vi "Configure Node Info.vi"(8 "error in (no error)":errorcluster, 11 "Volatus Core in":refnum<class "Volatus Core.lvclass">) -> (0 "error out":errorcluster, 3 "Volatus Core out":refnum<class "Volatus Core.lvclass">)   [LabVIEW 2020, in "Volatus.lvlib" / "Volatus Core.lvclass"]
uses:
  Volatus Core.lvclass
  C:/dev/lv20CE/relink/lv-volatus/Volatus/Module/Module.lvclass
  Volatus Core.lvclass/Volatus Core.ctl
  Module/Module.lvclass
  lv-vecto/Vecto/Node Config/Node Config.lvclass
  C:/dev/lv20CE/relink/lv-volatus/Volatus/Volatus Core/Volatus Core.lvclass
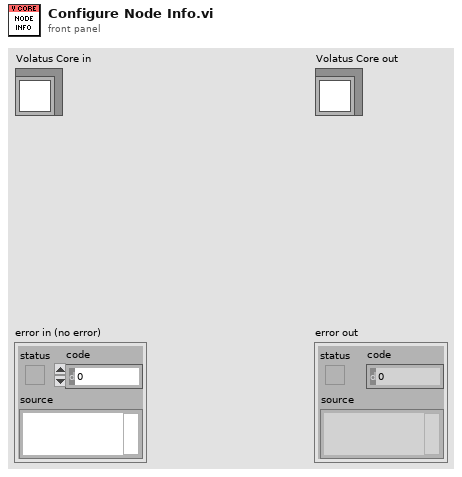
[diagram p1: front panel]
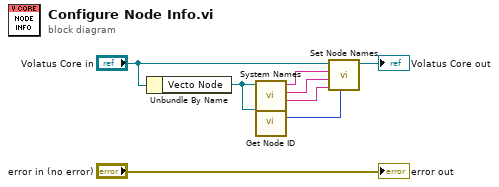
[diagram p0: block diagram]
diagram:
  n1 = Unbundle By Name("Volatus Core in") -> ("Vecto Node"=w2:refnum<class "Node Config.lvclass">)
  n2 = call "System Names.vi"("Node Config in"=w2) -> ("Name"=w4:string, "Cluster"=w5:string, "System"=w7:string)  [unwired: 8 in]
  n3 = call "Get Node ID.vi"("Node in"=w2) -> ("Node ID"=w1:u32)  [unwired: 8 in, 2 out]
  n4 = call "Set Node Names.vi"("Node ID"=w1, "Node"=w4, "Cluster"=w5, "System"=w7, "Module in"="Volatus Core in") -> ("Module out"=→"Volatus Core out":refnum<class "Volatus Core.lvclass">)  [unwired: 6 in]
  "error out" <- "error in (no error)"
